vi "MGI Delete Row[].vi"(8 "error in (no error)":errorcluster, 10 "Listbox row[] to delete":i32[](array[numeric]), 11 "MGI Error Handler in":refnum<class "MGI Error Reporter Dialog.lvclass">) -> (0 "error out":errorcluster, 3 "MGI Error Handler out":refnum<class "MGI Error Reporter Dialog.lvclass">)   [LabVIEW 2020, in "MGI Error Reporter Dialog.lvclass"]
doc: "Delete the error(s) in the specified Row[] from the History Listbox.\n\nAuthored by Shawn Walpole\nsupport@mooregoodideas.com\nwww.mooregoodideas.com\n\nCopyright (c) 2013, Moore Good Ideas, Inc.\n\nAll rights reserved.\n\nRedistribution and use in source and binary forms, with or without modification, are permitted provided that the following conditions are met:\n\n * Redistributions of source code must retain the above copyright notice, this list of conditions and the following disclaimer.\n * Redistributions in binary form must reproduce the above copyright notice, this list of conditions and the following disclaimer in the documentation and/or other materials provided with the distribution.\n * Neither the name of Moore Good Ideas, Inc. nor the names of its contributors may be used to endorse or promote products derived from this software without specific prior written permission.\n\nTHIS SOFTWARE IS PROVIDED BY THE COPYRIGHT HOLDERS AND CONTRIBUTORS \"AS IS\" AND ANY EXPRESS OR IMPLIED WARRANTIES, INCLUDING, BUT NOT LIMITED TO, THE IMPLIED WARRANTIES OF MERCHANTABILITY AND FITNESS FOR A PARTICULAR PURPOSE ARE DISCLAIMED. IN NO EVENT SHALL THE COPYRIGHT OWNER OR CONTRIBUTORS BE LIABLE FOR ANY DIRECT, INDIRECT, INCIDENTAL, SPECIAL, EXEMPLARY, OR CONSEQUENTIAL DAMAGES (INCLUDING, BUT NOT LIMITED TO, PROCUREMENT OF SUBSTITUTE GOODS OR SERVICES; LOSS OF USE, DATA, OR PROFITS; OR BUSINESS INTERRUPTION) HOWEVER CAUSED AND ON ANY THEORY OF LIABILITY, WHETHER IN CONTRACT, STRICT LIABILITY, OR TORT (INCLUDING NEGLIGENCE OR OTHERWISE) ARISING IN ANY WAY OUT OF THE USE OF THIS SOFTWARE, EVEN IF ADVISED OF THE POSSIBILITY OF SUCH DAMAGE."
uses:
  <userlib>/_MGI/Error Reporter/MGI Error Reporter Dialog/MGI Error Reporter Dialog.lvclass
  <userlib>/_MGI/Error Reporter/MGI Error Reporter Dialog/MGI Error Reporter Dialog.lvclass/MGI Error Reporter Dialog.ctl
  <userlib>/_MGI/Application Control/MGI Set Scrollbar/MGI Set Multicolumn Listbox Scrollbar.vi
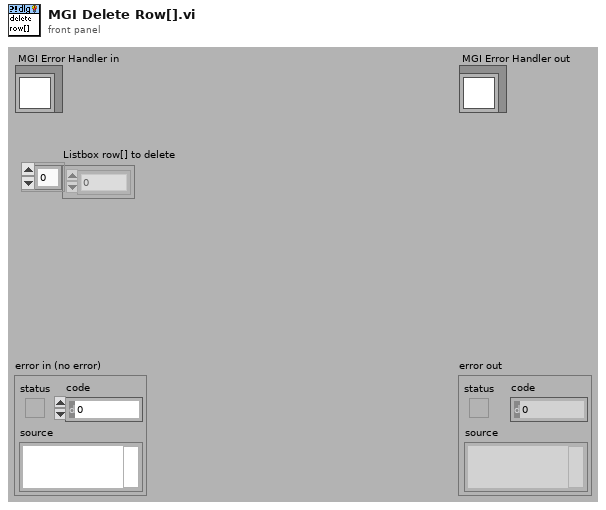
[diagram p1: front panel]
types:
  T1 = typedef "MGI Error Reporter Dialog.lvclass/MGI Dialog UI Refs Cluster.ctl" = cluster{"LB Ref":refnum<vi>, "Details Ref":refnum<vi>, "Caller Ring Ref":refnum<vi>, "Message Ref":refnum<vi>, "Clear Btn Ref":refnum<vi>}
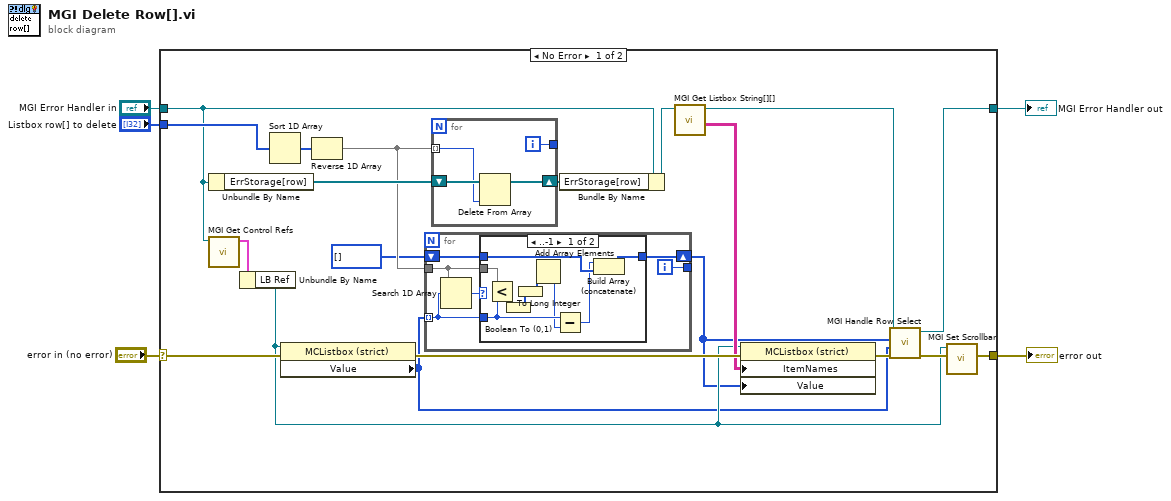
[diagram p0: block diagram]
diagram:
  n1 = case shown="No Error" "error in (no error)" {
    selector: "error in (no error)" -> [w19 w47]
    tunnel: [w16 w47] -> w4
    tunnel: [w17 w46] -> w2
    tunnel: "MGI Error Handler in" -> [w21 w46]
    tunnel: "Listbox row[] to delete" -> [w24 _]
    frame No Error {
      n2 = Unbundle By Name(w21) -> ("ErrStorage[row]"=w25:refnum<class "MGI ERD LB Row Base.lvclass">[])
      n3 = call <userlib>:"MGI Get Control Refs.vi"("MGI Error Dialog.lvclass"=w21) -> ("Refs"=w20:T1)  [unwired: 10 out]
      n4 = Unbundle By Name(w20) -> ("LB Ref"=w10:refnum<vi>)
      n5 = Sort 1D Array(array=w24) -> (sorted array=w23:i32[])
      n6 = property class="MCListbox (strict)"(reference=w10, error in=w19) -> (error out=w13:errorcluster, "Value"=w9:i32[])  [unwired: 1 out]
      n7 = Reverse 1D Array(array=w23) -> (reversed array=w8:i32[])
      n8 = for {
        shift-right: [w28] -> w6
        shift-left: i32[] [] ("Value") -> [w29]
        tunnel: w9 -> [w27] mode=indexing
        tunnel: w8 -> [w26]
        tunnel: [w31] -> _
        i -> [w31]
        n9 = Search 1D Array(1D array=w26, element=w27) -> (index of element=w30:i32)  [unwired: 1 out]
        n10 = case shown="..-1" w30 {
          tunnel: w29 -> [w40 w41]
          tunnel: [w39 w41] -> w28
          tunnel: w27 -> [w36 _]
          tunnel: w26 -> [w37 _]
          frame ..-1 {
            n11 = Less?(x=w37, y=w36) -> (x < y?=w35:bool[])
            n12 = Boolean To (0,1)(Boolean=w35) -> (0, 1=w34:i16[])
            n13 = To Long Integer(number=w34) -> (32bit integer=w33:i32[])
            n14 = Add Array Elements(numeric array=w33) -> (sum=w32:i32)
            n15 = Subtract(x=w36, y=w32) -> (x-y=w38:i32)
            n16 = Build Array (concatenate)(w38, w40) -> (w39:i32[])
          }
          frame 0.. {
          }
        }
      }
      n17 = for {
        shift-right: [w44] -> w22
        shift-left: w25 -> [w45]
        tunnel: w8 -> [w43] mode=indexing
        tunnel: [w42] -> _
        i -> [w42]
        n18 = Delete From Array(array=w45, index=w43) -> (array with subset deleted=w44:refnum<class "MGI ERD LB Row Base.lvclass">[])  [unwired: 1 in, 1 out]
      }
      n19 = Bundle By Name(cluster=w21, "ErrStorage[row]"=w22) -> (w15:refnum<class "MGI Error Reporter Dialog.lvclass">)
      n20 = call-dynamic "MGI Get Listbox String[][].vi"("MGI Error Dialog in"=w15) -> ("Error[Row][Err/Warn,Name,Time,Count]"=w11:string[][], "MGI Error Dialog out"=w14:refnum<class "MGI Error Reporter Dialog.lvclass">)  [unwired: 2 in, 7 out]
      n21 = property class="MCListbox (strict)"(reference=w10, error in=w13, "ItemNames"=w11, "Value"=w6) -> (error out=w12:errorcluster)  [unwired: 1 out]
      n22 = call-dynamic "MGI Handle Row Select.vi"("error in (no error)"=w12, "Old Selected[]"=w9, "Selected[]"=w6, "MGI Error Handler in"=w14) -> ("error out"=w18:errorcluster, "MGI Error Handler out"=w17:refnum<class "MGI Error Reporter Dialog.lvclass">)  [unwired: 6 out]
      n23 = call-poly <userlib>:"MGI Set Scrollbar.vi"("Error In"=w18, "Listbox Reference In"=w10) -> ("Error Out"=w16:errorcluster)  [unwired: 9 out]
    }
    frame Error {
    }
  }
  "error out" <- w4
  "MGI Error Handler out" <- w2
